vi "Set Up Dialog - Turbidity.vi"() -> ()   [LabVIEW 2012]
panel:
  out "Calibration Instructions":string="1. Connect the sensor to your myDAQ as shown in the diagram above.\n\n2. Set the sensor to Colorimeter mode. The sensor will only accept micro cuvette's.\n\n3. Prepare a clean cuvette with distilled water. The voltage should be 2.5V for all colors.\n\n4. Prepare another cuvette with black solution to block out all light. The output voltage should be 0V for all colors."
  # "iWorx - Turbidity - Set Up"
  # "Colorimeter (CTSN - 100)"
  # "iWorx"
  # "Sensor"
  # "CTSN - 100"
  # "myDAQ"
  # "Computer"
  # "Adaptor"
  # "Connection Diagram"
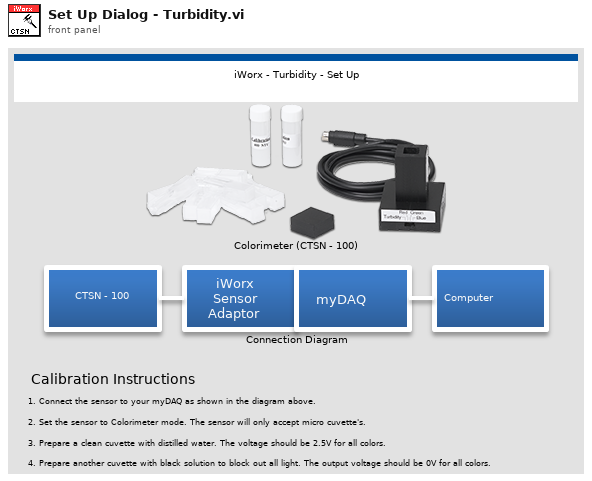
[diagram p1: front panel]
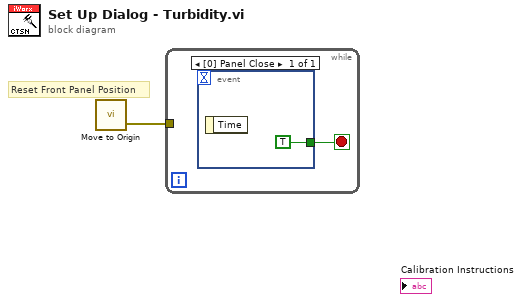
[diagram p0: block diagram]
diagram:
  # "Reset Front Panel Position"
  n1 = call "Move to Origin.vi"() -> ("Error Out"=w1:errorcluster)  [unwired: 3 in]
  n2 = while {
    tunnel: w1 -> [_]
    stop <- w2 stop-if-true
    n3 = event shown="[0] Panel Close" {
      selector: _ -> [_]
      dyn-events: _ -> [_]
      timeout: _ -> [_]
      tunnel: [TRUE] -> w2
      event Panel Close {
        n4 = event-data() -> ()  [unwired: 1 in, 1 out]
      }
    }
  }
